vi "TSF Manager Get Band Noise Settings.vi"(8 "error in (no error)":errorcluster, 11 "TSF Parser in":refnum<class "TSF Parser.lvclass">) -> (0 "error out":errorcluster, 2 "BandNoise Test Settings.lvlibp:Band Noise Test Settings.lvclass":refnum<class "Band Noise Test Settings.lvclass">, 3 "TSF Parser out":refnum<class "TSF Parser.lvclass">)   [LabVIEW 2016, in "TSF Parser.lvlib" / "TSF Parser.lvclass"]
uses:
  TSF Parser.lvclass
  Plugins/Test Settings/BandNoise Test Settings.lvlibp/Band Noise Test Settings.lvclass
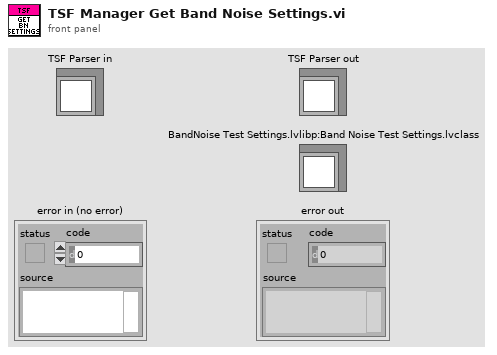
[diagram p1: front panel]
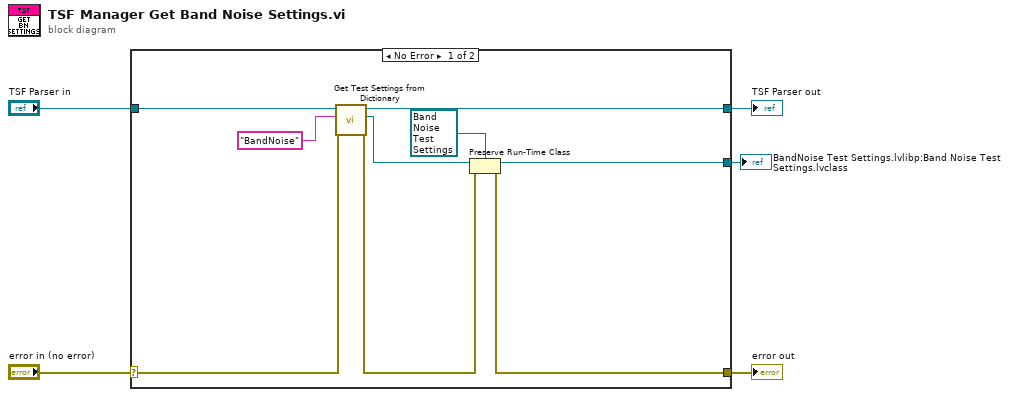
[diagram p0: block diagram]
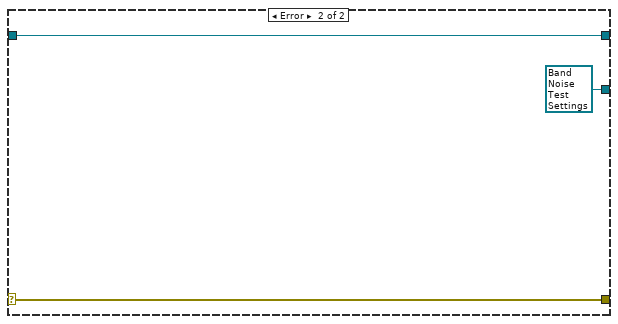
[diagram p2: hidden frame]
diagram:
  n1 = case shown="No Error" "error in (no error)" {
    selector: "error in (no error)" -> [w12 w17]
    tunnel: [w6 w17] -> w4
    tunnel: [w13 w16] -> w2
    tunnel: "TSF Parser in" -> [w14 w16]
    tunnel: [w8 refnum<class "Band Noise Test Settings.lvclass"> refnum ("BandNoise Test Settings.lvlibp:Band Noise Test Settings.lvclass")] -> w1
    frame No Error {
      n2 = call "Get Test Settings from Dictionary.vi"("error in (no error)"=w12, "name"="BandNoise", "TSF Parser in"=w14) -> ("error out"=w7:errorcluster, "ITestSettings Out"=w10:refnum<class "ITestSettings.lvclass">, "TSF Parser out"=w13:refnum<class "TSF Parser.lvclass">)  [unwired: 6 in]
      n3 = Preserve Run-Time Class(object in=w10, error in=w7, 2:refnum<class "Band Noise Test Settings.lvclass"> refnum ("BandNoise Test Settings.lvlibp:Band Noise Test Settings.lvclass")) -> (object out=w8:refnum<class "Band Noise Test Settings.lvclass">, error out=w6:errorcluster)
    }
    frame Error {
    }
  }
  "error out" <- w4
  "TSF Parser out" <- w2
  "BandNoise Test Settings.lvlibp:Band Noise Test Settings.lvclass" <- w1
